vi "AutoFilename.vi"(0 "File Path Parameter":T7={"Filename Prefix"="MyData", "Extension"=enum."±Field", "Suffix"="", "Current Path"=path "/opticsmac/Users/Data"}, 7 "File Info Parameter":T1={"FilePath"=path "/Opticsmac/Documents/Data", "Field (T)"=55.0, "Temperature (K)"=77.0, "X-Axis"=enum."nm", "Center nm"=600.0, "Current Grating Density"=enum."600", "CCD Parameters"={"Exposure Time (s)"=0.2, "Offset"=0.0, "BkgrdCrct"=FALSE, "Shutter"=FALSE, "Mode"=enum."Regular", "Repetition"=4, "dt or s"=0.0}, "Operation Mode"=enum."NML Data Acquisition", "Exp Index"=0, "Index_repetition"=0, "Index"=0, "Current Detector"=enum."CCD-1024x256"} {"CCD Parameters"."dt or s" format="%#.6f"; "CCD Parameters"."Repetition" min=1; "CCD Parameters"."Offset" format="%#.2f"; "CCD Parameters"."Exposure Time (s)" min=0.02 max=6000.0 format="%#.2f"; "Center nm" format="%.2f"; "Temperature (K)" format="%.2f"; "Field (T)" format="%.2f"}, 13 "Format String":string[](array[string])=["%+06.2fT", "%04.1fK"]) -> (4 "File path Output":path, 8 "FileNameOut":string="MyDataA-23.46T04.2K", 15 "File Info Parameter Output":T1={"FilePath"=path "/Opticsmac/Documents/Data", "Field (T)"=55.0, "Temperature (K)"=77.0, "X-Axis"=enum."nm", "Center nm"=600.0, "Current Grating Density"=enum."600", "CCD Parameters"={"Exposure Time (s)"=0.2, "Offset"=0.0, "BkgrdCrct"=FALSE, "Shutter"=FALSE, "Mode"=enum."Regular", "Repetition"=4, "dt or s"=0.0}, "Operation Mode"=enum."NML Data Acquisition", "Exp Index"=0, "Index_repetition"=0, "Index"=0, "Current Detector"=enum."CCD-1024x256"} {"CCD Parameters"."dt or s" format="%#.6f"; "CCD Parameters"."Repetition" min=1; "CCD Parameters"."Offset" format="%#.2f"; "CCD Parameters"."Exposure Time (s)" min=0.02 max=6000.0 format="%#.2f"; "Center nm" format="%.2f"; "Temperature (K)" format="%.2f"; "Field (T)" format="%.2f"})   [LabVIEW 2021]
uses:
  Globals and TypeDefs/Type Definitions.llb/FilePathParameter.ctt
  Globals and TypeDefs/Type Definitions.llb/FileInfoParameter.ctt
  Globals and TypeDefs/Type Definitions.llb/Wavelength Unit.ctt
  Globals and TypeDefs/Type Definitions.llb/McPherson Grating Density.ctl
  Globals and TypeDefs/Type Definitions.llb/CCDParameter.ctt
  Globals and TypeDefs/Type Definitions.llb/OperationMode.ctt
  Globals and TypeDefs/Type Definitions.llb/ListOfDetectors.ctt
  X-Axis Converter.llb/X-Point Converter.vi
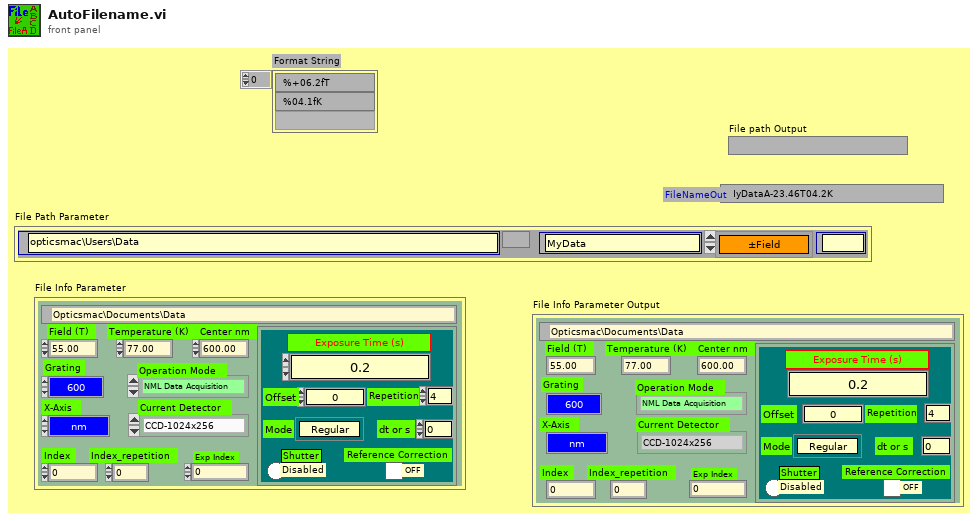
[diagram p1: front panel]
types:
  T1 = typedef "FileInfoParameter.ctt" = cluster{"FilePath":path, "Field (T)":dbl, "Temperature (K)":dbl, "X-Axis":T2, "Center nm":dbl, "Current Grating Density":T3, "CCD Parameters":T4, "Operation Mode":T5, "Exp Index":u32, "Index_repetition":u16, "Index":u16, "Current Detector":T6}
  T2 = typedef "Wavelength Unit.ctt" = enum8{"Point", "nm", "eV", "meV", "cm_1"}
  T3 = typedef "McPherson Grating Density.ctl" = enum8{"150", "300", "600", "1200", "1800"}
  T4 = typedef "CCDParameter.ctt" = cluster{"Exposure Time (s)":dbl, "Offset":dbl, "BkgrdCrct":bool, "Shutter":bool, "Mode":enum8{"Regular", "OverExp Cor", "SpikeRemove", "ForCalibration"}, "Repetition":u16, "dt or s":dbl}
  T5 = typedef "OperationMode.ctt" = enum16{"Standby", "CCD Single Shot", "CCD Sequence Shots", "CCD Custom Shots", "CCD Reference Shot", "Step Scanning ", "Time Scanning", "NML Data Acquisition"}
  T6 = typedef "ListOfDetectors.ctt" = enum8{"CCD-1024x256", "InGaAs PDA-1024x1", "CCD-1340x400", "Ge Single Channel", "Si Single Channel", "PMT Single Channel"}
  T7 = typedef "FilePathParameter.ctt" = cluster{"Filename Prefix":string, "Extension":enum16{"none", "\".001\",\".002\", ...", "001 (No dot)", "±Field", "pField nField", "Temperature", "Wavelength", "T(K)±H(T)", "(nm)T(K)±H(T)", "User Defined"}, "Suffix":string, "Current Path":path}
  T8 = enum16{"DOS field", "\".001\",\".002\", ...", "001 (No dot)", "±Field", "pField nField", "Temperature", "Wavelength", "T(K)±H(T)", "(nm)T(K)±H(T)", "User Defined"}
  T9 = enum16{"none", "\".001\",\".002\", ...", "001 (No dot)", "±Field", "pField nField", "Temperature", "Wavelength", "T(K)±H(T)", "(nm)T(K)±H(T)", "User Defined"}
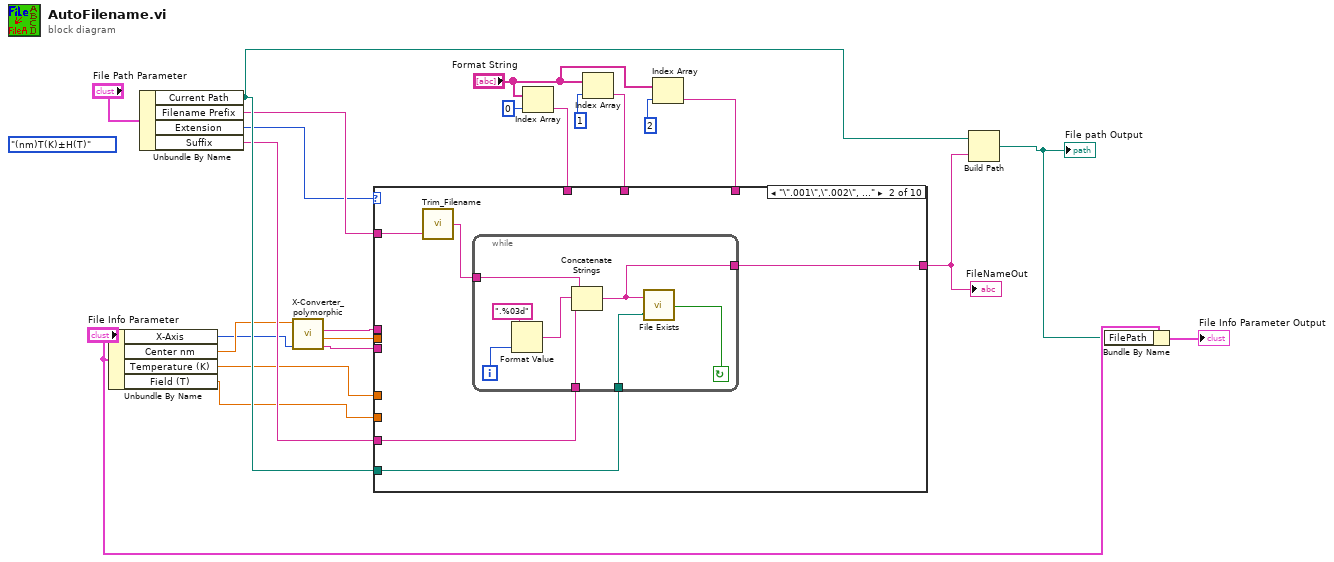
[diagram p0: block diagram]
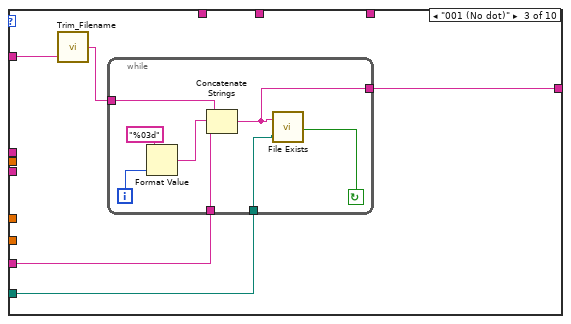
[diagram p3: hidden frame]
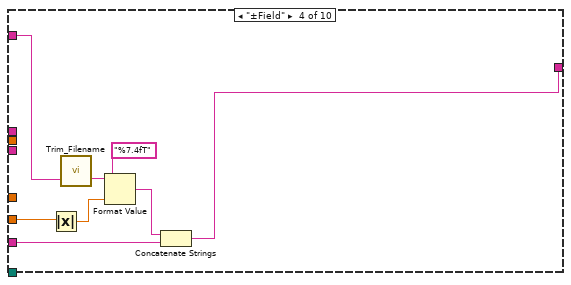
[diagram p4: hidden frame]
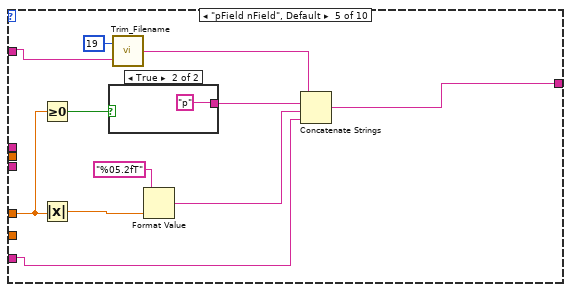
[diagram p5: hidden frame]
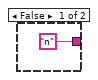
[diagram p6: hidden frame]
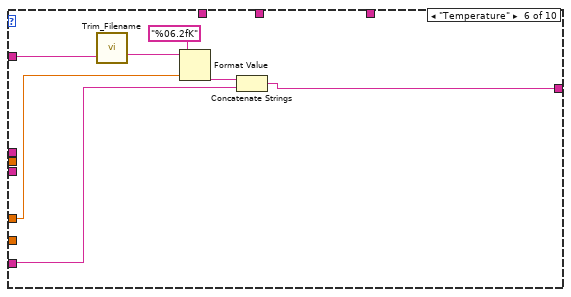
[diagram p7: hidden frame]
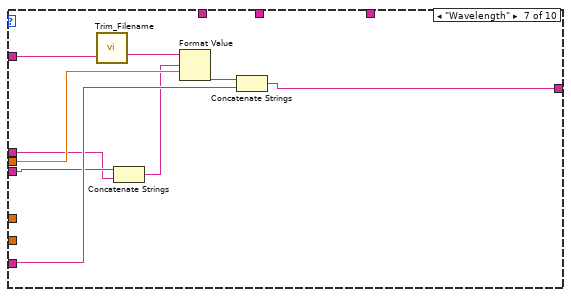
[diagram p8: hidden frame]
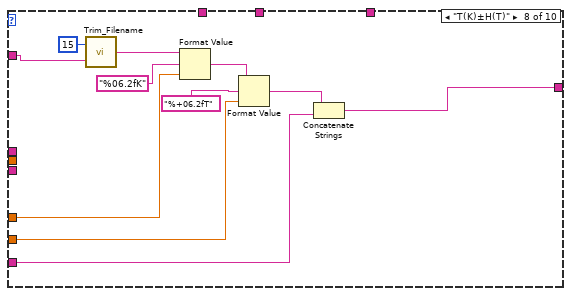
[diagram p9: hidden frame]
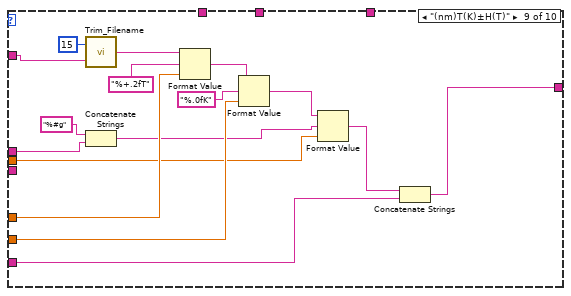
[diagram p10: hidden frame]
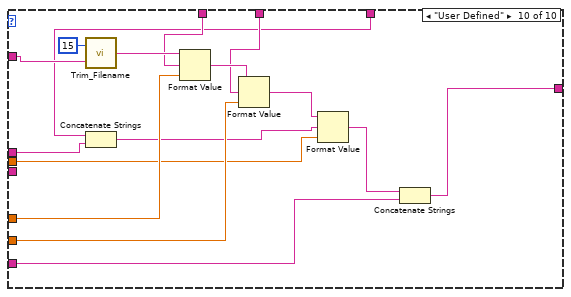
[diagram p11: hidden frame]
diagram:
  (unwired) T8."(nm)T(K)±H(T)" ("Extension")
  n1 = Unbundle By Name("File Info Parameter") -> ("X-Axis"=w7:T2, "Center nm"=w8:dbl, "Temperature (K)"=w14:dbl, "Field (T)"=w13:dbl)
  n2 = Unbundle By Name("File Path Parameter") -> ("Current Path"=w17:path, "Filename Prefix"=w16:string, "Extension"=w9:T9, "Suffix"=w15:string)
  n3 = call-poly "X-Converter_polymorphic.vi"("X-Axis Unit"=w7, "X-Axis input"=w8) -> ("UnitFormatString"=w5:string, "X-Axis Output"=w6:dbl, "X-Axis Unit String"=w4:string)  [unwired: 3 in, 1 out]
  n4 = Index Array(array="Format String", index=0) -> (element=w21:string)
  n5 = Index Array(array="Format String", index=1) -> (element=w20:string)
  n6 = Index Array(array="Format String", index=2) -> (element=w1:string)
  n7 = case shown="\"\\\".001\\\",\\\".002\\\", ...\"" w9 {
    tunnel: w16 -> [w24 w29 w42 w53 w61 w74 w84 w92 w109 w125]
    tunnel: w14 -> [_ _ _ _ w67 w72 _ w97 w113 w129]
    tunnel: w13 -> [_ _ _ w51 _ _ _ w95 w111 w127]
    tunnel: [w24 w25 w38 w55 w65 w75 w85 w98 w114 w130] -> w19
    tunnel: w15 -> [_ w27 w40 w56 w62 w76 w86 w93 w110 w126]
    tunnel: w17 -> [_ w26 w39 _ _ _ _ _ _ _]
    tunnel: w21 -> [_ _ _ _ _ _ _ _ _ w117]
    tunnel: w20 -> [_ _ _ _ _ _ _ _ _ w116]
    tunnel: w6 -> [_ _ _ _ _ _ w82 _ w104 w120]
    tunnel: w5 -> [_ _ _ _ _ _ w81 _ _ _]
    tunnel: w4 -> [_ _ _ _ _ _ w80 _ w102 w119]
    tunnel: w1 -> [_ _ _ _ _ _ _ _ _ w115]
    frame "none" {
    }
    frame "\".001\",\".002\", ..." {
      n8 = call "Trim_Filename.vi"("Input string"=w29) -> ("output string"=w28:string)  [unwired: 1 in]
      n9 = while {
        tunnel: [w32] -> w25
        tunnel: w26 -> [w31]
        tunnel: w27 -> [w33]
        tunnel: w28 -> [w35]
        i -> [w36]
        stop <- w30 continue-if-true
        n10 = Format Value(format string=".%03d", value (0)=w36) -> (output string=w34:string)  [unwired: 1 in]
        n11 = Concatenate Strings(w35, w34, w33) -> (w32:string)
        n12 = call "File Exists.vi"("Dir Path"=w31, "FILESPEC"=w32) -> (0:w30:bool)
      }
    }
    frame "001 (No dot)" {
      n13 = call "Trim_Filename.vi"("Input string"=w42) -> ("output string"=w41:string)  [unwired: 1 in]
      n14 = while {
        tunnel: [w44] -> w38
        tunnel: w39 -> [w43]
        tunnel: w40 -> [w46]
        tunnel: w41 -> [w48]
        i -> [w49]
        stop <- w45 continue-if-true
        n15 = Format Value(format string="%03d", value (0)=w49) -> (output string=w47:string)  [unwired: 1 in]
        n16 = Concatenate Strings(w48, w47, w46) -> (w44:string)
        n17 = call "File Exists.vi"("Dir Path"=w43, "FILESPEC"=w44) -> (0:w45:bool)
      }
    }
    frame "±Field" {
      n18 = Absolute Value(x=w51) -> (abs(x)=w52:dbl)
      n19 = call "Trim_Filename.vi"("Input string"=w53) -> ("output string"=w54:string)  [unwired: 1 in]
      n20 = Format Value(string ("")=w54, format string="%7.4fT", value (0)=w52) -> (output string=w57:string)
      n21 = Concatenate Strings(w57, w56) -> (w55:string)
    }
    frame "pField nField", Default {
      n22 = Greater Or Equal To 0?(x=w67) -> (x >= 0?=w68:bool)
      n23 = Absolute Value(x=w67) -> (abs(x)=w66:dbl)
      n24 = case shown="True" w68 {
        tunnel: ["n" "p"] -> w64
        frame False {
        }
        frame True {
        }
      }
      n25 = call "Trim_Filename.vi"("Input string"=w61, "length"=19) -> ("output string"=w60:string)
      n26 = Format Value(format string="%05.2fT", value (0)=w66) -> (output string=w63:string)  [unwired: 1 in]
      n27 = Concatenate Strings(w60, w64, w63, w62) -> (w65:string)
    }
    frame "Temperature" {
      n28 = call "Trim_Filename.vi"("Input string"=w74) -> ("output string"=w73:string)  [unwired: 1 in]
      n29 = Format Value(string ("")=w73, format string="%06.2fK", value (0)=w72) -> (output string=w77:string)
      n30 = Concatenate Strings(w77, w76) -> (w75:string)
    }
    frame "Wavelength" {
      n31 = call "Trim_Filename.vi"("Input string"=w84) -> ("output string"=w83:string)  [unwired: 1 in]
      n32 = Concatenate Strings(w81, w80) -> (w79:string)
      n33 = Format Value(string ("")=w83, format string=w79, value (0)=w82) -> (output string=w87:string)
      n34 = Concatenate Strings(w87, w86) -> (w85:string)
    }
    frame "T(K)±H(T)" {
      n35 = call "Trim_Filename.vi"("Input string"=w92, "length"=15) -> ("output string"=w91:string)
      n36 = Format Value(string ("")=w91, format string="%06.2fK", value (0)=w97) -> (output string=w96:string)
      n37 = Format Value(string ("")=w96, format string="%+06.2fT", value (0)=w95) -> (output string=w94:string)
      n38 = Concatenate Strings(w94, w93) -> (w98:string)
    }
    frame "(nm)T(K)±H(T)" {
      n39 = call "Trim_Filename.vi"("Input string"=w109, "length"=15) -> ("output string"=w108:string)
      n40 = Concatenate Strings("%#g", w102) -> (w101:string)
      n41 = Format Value(string ("")=w108, format string="%+.2fT", value (0)=w113) -> (output string=w112:string)
      n42 = Format Value(string ("")=w112, format string="%.0fK", value (0)=w111) -> (output string=w106:string)
      n43 = Format Value(string ("")=w106, format string=w101, value (0)=w104) -> (output string=w105:string)
      n44 = Concatenate Strings(w105, w110) -> (w114:string)
    }
    frame "User Defined" {
      n45 = call "Trim_Filename.vi"("Input string"=w125, "length"=15) -> ("output string"=w124:string)
      n46 = Concatenate Strings(w115, w119) -> (w118:string)
      n47 = Format Value(string ("")=w124, format string=w117, value (0)=w129) -> (output string=w128:string)
      n48 = Format Value(string ("")=w128, format string=w116, value (0)=w127) -> (output string=w122:string)
      n49 = Format Value(string ("")=w122, format string=w118, value (0)=w120) -> (output string=w121:string)
      n50 = Concatenate Strings(w121, w126) -> (w130:string)
    }
  }
  "FileNameOut" <- w19
  n51 = Build Path(base path=w17, name or relative path=w19) -> (appended path=w11:path)
  "File path Output" <- w11
  n52 = Bundle By Name(cluster="File Info Parameter", "FilePath"=w11) -> (→"File Info Parameter Output":T1)
